vi "Video Extensometer.vi"() -> ()   [LabVIEW 2013]
uses:
  <vilib>/userdefined/High Color/IMAQdx.ctl
  <vilib>/vision/driver/IMAQdx.llb/IMAQdx Buffer Number Mode.ctl
  <vilib>/Analysis/baseanly.llb/Mean (DBL).vi
  Instance           1 30Saved   Shear-C273-with-Unload .vi
  Instance           4 30Saved   Shear-C273-with-Unload .vi
  <vilib>/vision/driver/NI_Vision_Acquisition_Software.lvlib
  <resource>/objmgr/imaqdx.rc
  <vilib>/Analysis/NI_AALBase.lvlib
panel:
  in  "Timed \nAcquisition":bool
  in  "Data \nAcquisition \nInterval (s)":dbl=1.0 min=0.1 max=60.0
  out "Image":T1(plugin-control)
  out "Time":u32
  in  "Shutter":dbl(slide)=20.0 min=0.0 max=4095.0 step=1.0 scale=4.095..4095.0 scale format="%#.0f"
  in  "Brightness":dbl(slide)=200.0 min=0.0 max=255.0 step=1.0 scale=0.0..255.0
  in  "Gain":dbl(slide)=702.0 min=350.0 max=1000.0 step=1.0 scale=350.0..1000.0
  in  "Video Mode Top":u32(ring)=47 items=["320x240 Color"=4, "640x480 Mono8"=9, "640x480 Mono16"=19, "640x480 Color"=14, "800x600 Mono8"=21, "800x600 Mono16"=27, "800x600 Color"=24, "1024x768 Mono8"=30, "1024x768 Mono16"=36, "1024x768 Color"=33, "1280x960 Mono8"=40, "1280x960 Mono16"=46, "1280x960 Color"=43, "1388x1038 Color"=47, "1388x1038 Mono"=48]
  in  "Session In Top View":T2="cam2"
  in  "Capture Current Image":bool
  in  "Begin Loading":bool
  out "Displacement (mm)":dbl
  in  "Pause":bool
  out "Crosshead Displacement":cluster{dbl[], dbl[]}(graph)
  in  "Unload \nVelocity":dbl=20.0
  in  "Unload":bool
  in  "Load Cell\nSelection":enum16{"300lb", "5lb", "50lb", "100lb"}(ring)
  in  "Distance to Travel (microns) \nup is positive":dbl=250000.0
  in  "Velocity (microns/sec)":dbl=5.0
  in  "Filename":string
  in  "Storage Directory":path=path "D:/AMS_Users_2014_2015/Michael Rossol"
  in  "Material":string
  in  "Stop":bool
  # "Top View Camera"
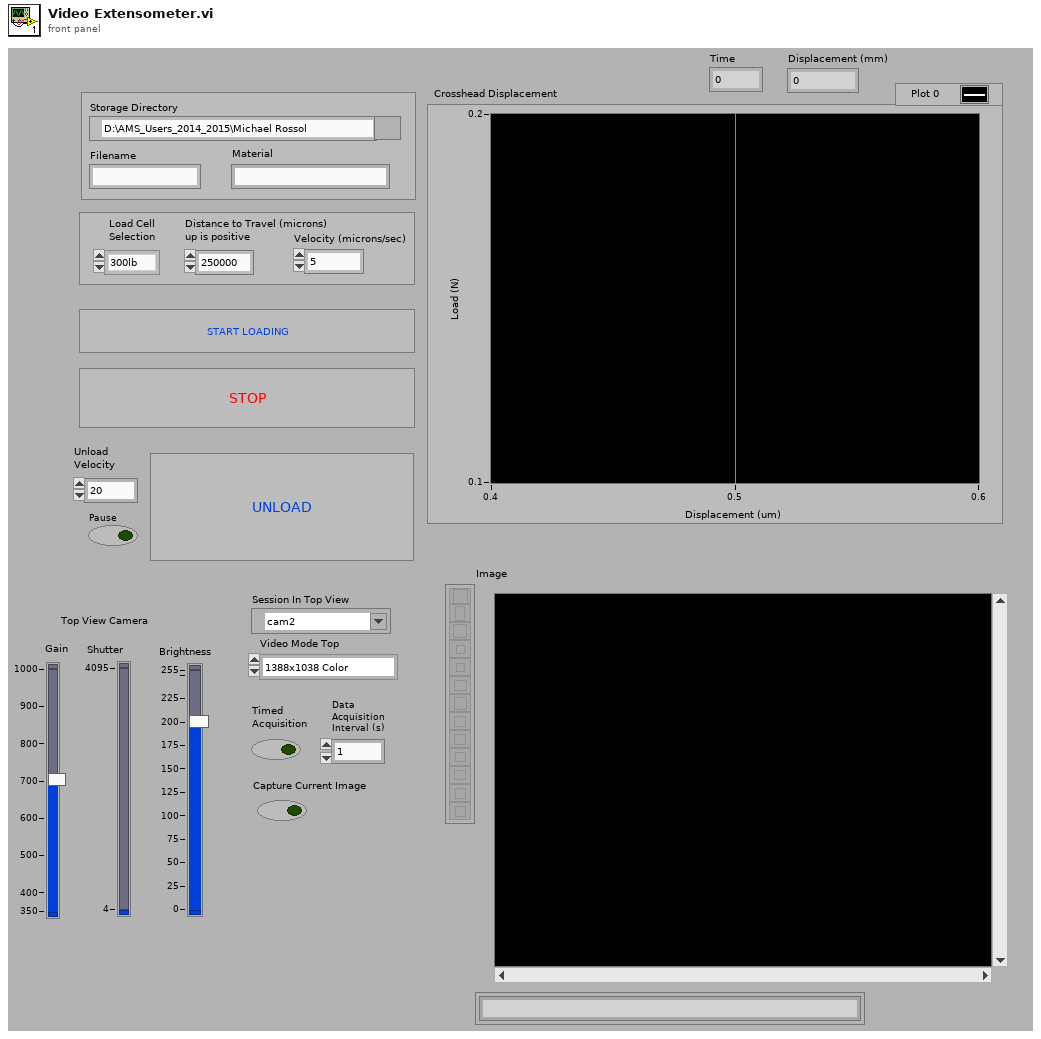
[diagram p1: front panel]
types:
  T1 = typedef "IMAQ Image.ctl" = refnum<image>
  T2 = typedef "IMAQdx.ctl" = refnum<k21>
  T3 = typedef "Image Type" = u32
  T4 = enum16{"open", "open or create", "create or replace", "create", "open (read only)"}
  T5 = typedef "NI_Vision_Acquisition_Software.lvlib/IMAQdx Buffer Number Mode.ctl" = enum32{"Next", "Last", "Buffer Number"}
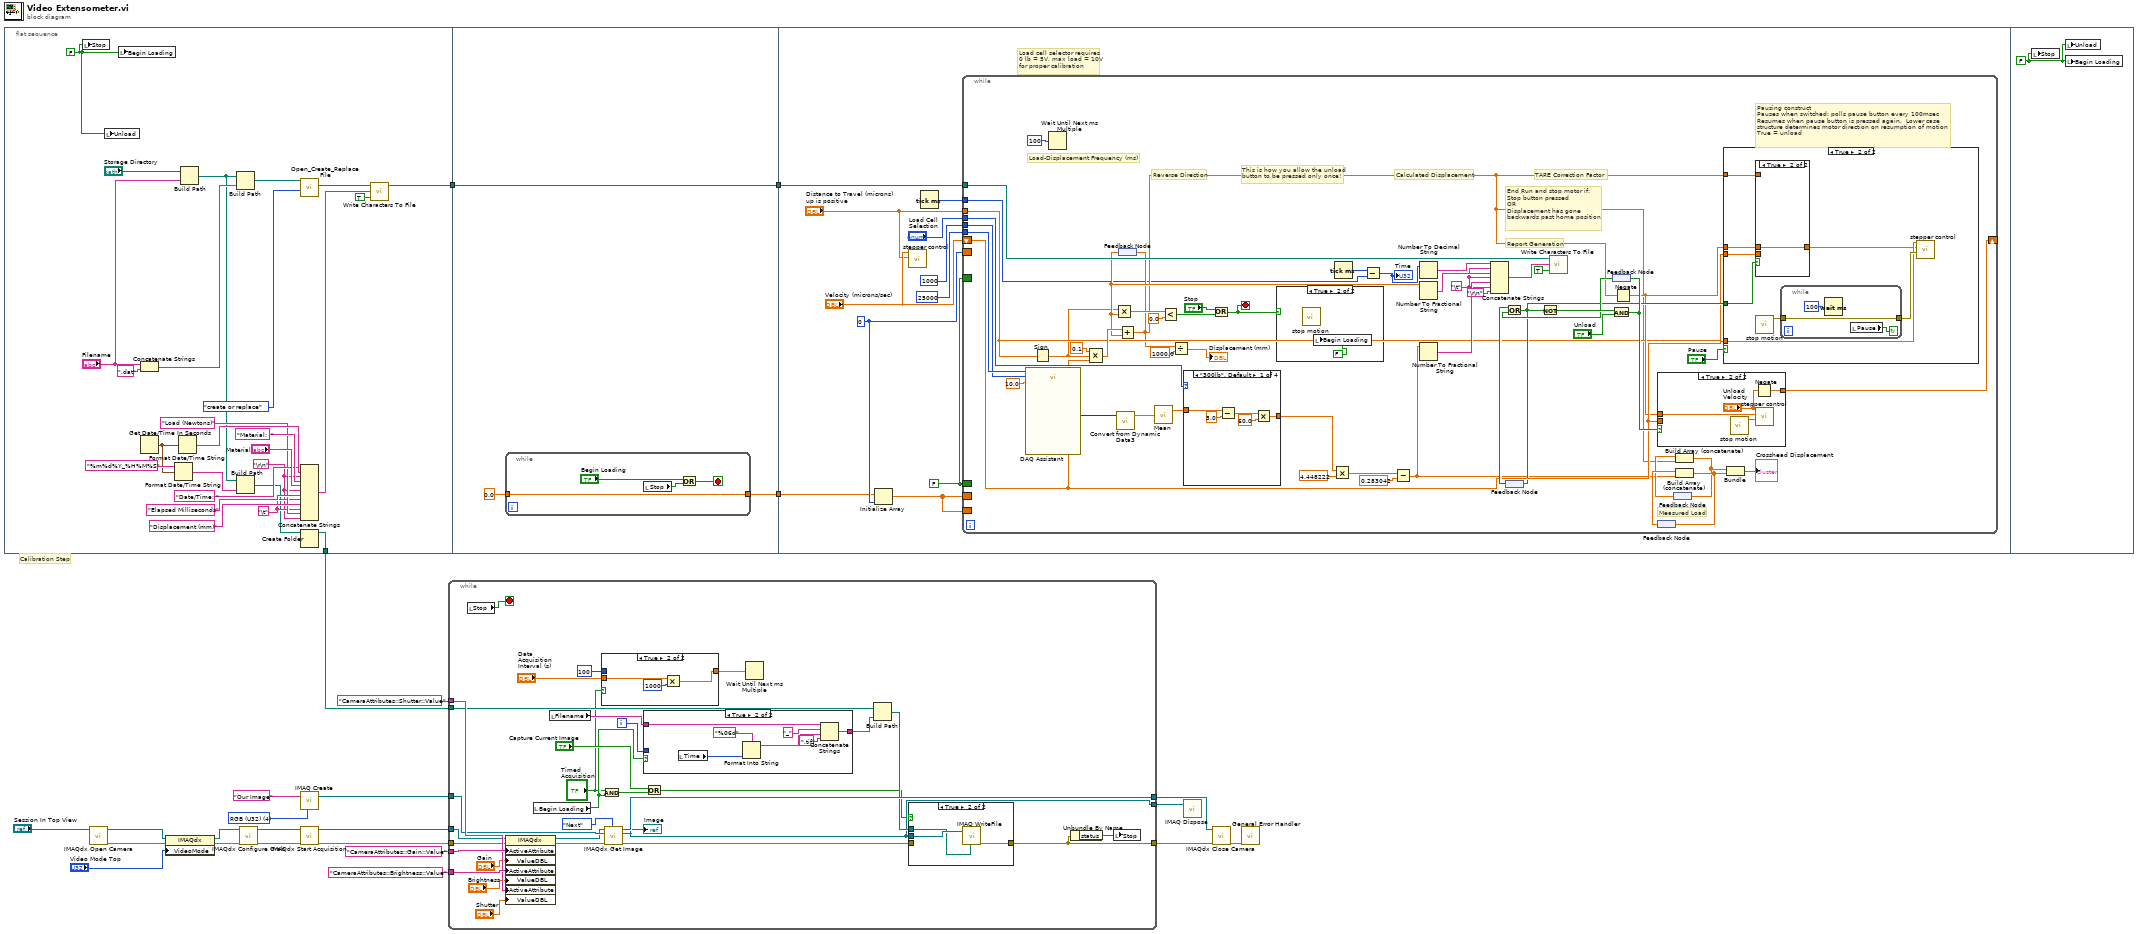
[diagram p0: block diagram]
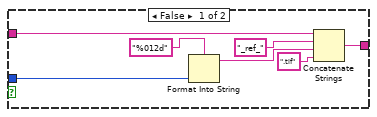
[diagram p2: hidden frame]
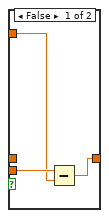
[diagram p6: hidden frame]
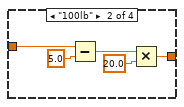
[diagram p9: hidden frame]
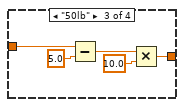
[diagram p10: hidden frame]
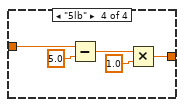
[diagram p11: hidden frame]
diagram:
  w17 = T3 4 items=["Grayscale (U8)", "Grayscale (I16)", "Grayscale (SGL)", "Complex (CSG)", "RGB (U32)", "HSL (U32)", "RGB (U64)"] ("Image Type")
  # "Calibration Step"
  n1 = flat-sequence {
    tunnel: [w41] -> w24
    tunnel: [w28] -> w1
    tunnel: w24 -> [w53]
    tunnel: [w53] -> w23
    tunnel: [w51] -> w22
    tunnel: w23 -> [w63]
    tunnel: w22 -> [w59]
    frame #0 {
      w35 = "\t"
      w25 = FALSE ("Begin Loading")
      w32 = "\r\n"
      n2 = local write "Stop"(w25) -> ()
      n3 = local write "Unload"(w25) -> ()
      n4 = local write "Begin Loading"(w25) -> ()
      n5 = Get Date/Time In Seconds() -> (seconds since 1Jan1904=w27:timestamp)
      n6 = Concatenate Strings("Filename", ".dat") -> (w47:string)
      n7 = Format Date/Time String(time format string (%c)="%m%d%Y_%H%M%S", seconds (now)=w27) -> (date/time string=w26:string)  [unwired: 1 in]
      n8 = Format Date/Time String(seconds (now)=w27) -> (date/time string=w43:string)  [unwired: 2 in]
      n9 = Build Path(base path="Storage Directory", name or relative path="Filename") -> (appended path=w30:path)
      n10 = Build Path(base path=w30, name or relative path=w47) -> (appended path=w40:path)
      n11 = Build Path(base path=w30, name or relative path=w26) -> (appended path=w29:path)
      n12 = call <vilib>:"Open_Create_Replace File.vi"("function (open:0)"=T4."create or replace", "file path"=w40) -> ("new file path"=w49:path)  [unwired: 6 in, 3 out]
      n13 = Concatenate Strings("Date/Time: ", w43, w32, "Material:  ", "Material", w32, "Elapsed Milliseconds" ("string"), w35, "Displacement (mm)" ("string"), w35, "Load (Newtons)" ("string"), w32) -> (w45:string)
      n14 = Create Folder(path (use dialog)=w29) -> (created path=w28:path)  [unwired: 2 in, 2 out]
      n15 = call <vilib>:"Write Characters To File.vi"("append to file? (new file:F)"=TRUE, "character string"=w45, "file path (dialog if empty)"=w49) -> ("new file path (Not A Path if cancelled)"=w41:path)  [unwired: 2 in]
    }
    frame #1 {
      n16 = while {
        tunnel: [w57] -> w51
        tunnel: 0.0 ("element") -> [w57]
        stop <- w55 stop-if-true
        n17 = local read "Stop"() -> (w54:bool)
        n18 = Or(x="Begin Loading", y=w54) -> (x .or. y?=w55:bool)
      }
    }
    frame #2 {
      w68 = FALSE
      w67 = 0 ("dimension size")
      # "Load cell selector requires\n0 lb = 5V, max load = 10V\nfor proper calibration"
      n19 = Initialize Array(w59, w67) -> (w66:dbl[])
      n20 = call "stepper control.vi"("Distance to Travel (microns) \nup  is positive"="Distance to Travel (microns) \nup is positive", "Velocity (microns/sec)"="Velocity (microns/sec)") -> ()  [unwired: 9 in, 1 out]
      n21 = Tick Count (ms)() -> (millisecond timer value=w58:u32)
      n22 = while {
        tunnel: "Load Cell\nSelection" -> [w119]
        tunnel: w63 -> [w109]
        shift-right: [w108] -> _
        shift-left: "Velocity (microns/sec)" -> [w93]
        tunnel: "Distance to Travel (microns) \nup is positive" -> [w90]
        border: w66 -> [_]
        border: w67 -> [_]
        border: w66 -> [_]
        border: w68 -> [_]
        border: w68 -> [_]
        tunnel: 25000 ("Sampling Rate") -> [w84]
        tunnel: 1000 ("Sampling Rate") -> [w83]
        tunnel: w58 -> [w72]
        stop <- w107 stop-if-true
        w74 = "\t"
        # "Load-Displacement Frequency (ms)"
        # "TARE Correction Factor"
        # "Pausing construct\nPauses when switched; polls pause button every 100msec\nResumes when pause button is pressed again.  Lower case\nstructure determines motor direction on resumption of motion\nTrue = unload"
        # "This is how you allow the unload\nbutton to be pressed only once!"
        # "Reverse Direction"
        # "Calculated Displacement"
        # "Measured Load"
        # "End Run and stop motor if:\nStop button pressed\nOR\nDisplacement has gone \nbackwards past home position"
        # "Report Generation"
        n23 = call "DAQ Assistant"("rate"=w84, "number of samples"=w83, "timeout (s)"=10.0 ("timeout (sec)")) -> ("data"=w85:dynamicdata)  [unwired: 14 in, 2 out]
        n24 = Sign(1:w90) -> (0:w87:dbl)
        n25 = Wait Until Next ms Multiple(millisecond multiple=100 ("Loop Timing")) -> ()  [unwired: 1 out]
        n26 = Compound Arithmetic op=MULTIPLY(0.1 ("x"), w87, w93) -> (w104:dbl)
        n27 = call "Convert from Dynamic Data3"("Dynamic Data Type"=w85) -> ("Array"=w82:dbl[])  [unwired: 3 in]
        n28 = feedback #1() -> (w88:dbl)
        n29 = Multiply(x=w87, y=w88) -> (x*y=w89:dbl)
        n30 = Add(x=w104, y=w88) -> (x+y=w77:dbl)
        n31 = feedback-in #1(w77) -> ()
        n32 = call-poly <vilib>:"Mean.vi"("X"=w82) -> ("mean"=w81:dbl)  [unwired: 1 out]
        n33 = Less?(x=w89, y=0.0) -> (x < y?=w106:bool)
        n34 = Divide(x=w77, y=1000.0 ("timeout (sec)")) -> (x/y=→"Displacement (mm)":dbl)
        n35 = case shown="\"300lb\", Default" w119 {
          tunnel: w81 -> [w144 w148 w156 w161]
          tunnel: [w146 w147 w155 w160] -> w117
          frame "300lb", Default {
            n36 = Subtract(x=w144, y=5.0) -> (x-y=w142:dbl)
            n37 = Multiply(x=w142, y=60.0) -> (x*y=w146:dbl)
          }
          frame "100lb" {
            n38 = Subtract(x=w148, y=5.0) -> (x-y=w150:dbl)
            n39 = Multiply(x=w150, y=20.0) -> (x*y=w147:dbl)
          }
          frame "50lb" {
            n40 = Subtract(x=w156, y=5.0) -> (x-y=w153:dbl)
            n41 = Multiply(x=w153, y=10.0) -> (x*y=w155:dbl)
          }
          frame "5lb" {
            n42 = Subtract(x=w161, y=5.0) -> (x-y=w158:dbl)
            n43 = Multiply(x=w158, y=1.0) -> (x*y=w160:dbl)
          }
        }
        n44 = Or(x="Stop", y=w106) -> (x .or. y?=w107:bool)
        n45 = case shown="True" w107 {
          frame False {
          }
          frame True {
            n46 = call "stop motion.vi"() -> ()  [unwired: 11 in, 1 out]
            n47 = local write "Begin Loading"(FALSE ("Begin Loading")) -> ()
          }
        }
        n48 = Multiply(x=w117, y=4.448222) -> (x*y=w80:dbl)
        n49 = Tick Count (ms)() -> (millisecond timer value=w71:u32)
        n50 = Subtract(x=w71, y=w72) -> (x-y=w70:u32)
        "Time" <- w70
        n51 = Subtract(x=w80, y=0.283042) -> (x-y=w78:dbl)
        n52 = Number To Decimal String(number=w70) -> (decimal integer string=w73:string)  [unwired: 1 in]
        n53 = Number To Fractional String(number=w88) -> (F-format string=w111:string)  [unwired: 3 in]
        n54 = Number To Fractional String(number=w78) -> (F-format string=w110:string)  [unwired: 3 in]
        n55 = Concatenate Strings(w73, w74, w111, w74, w110, w74, "\r\n") -> (w113:string)
        n56 = feedback #2() -> (w103:bool)
        n57 = call <vilib>:"Write Characters To File.vi"("append to file? (new file:F)"=TRUE, "character string"=w113, "file path (dialog if empty)"=w109) -> ()  [unwired: 2 in, 1 out]
        n58 = feedback #3() -> (w101:bool)
        n59 = Or(x=w103, y=w101) -> (x .or. y?=w92:bool)
        n60 = feedback-in #2(w92) -> ()
        n61 = Not(x=w92) -> (.not. x?=w102:bool)
        n62 = And(x=w102, y="Unload") -> (x .and. y?=w99:bool)
        n63 = feedback-in #3(w99) -> ()
        n64 = Negate(x=w77) -> (-x=w91:dbl)
        n65 = case shown="True" w99 {
          tunnel: w91 -> [_ w140]
          tunnel: [w136 w139] -> w108
          tunnel: w93 -> [w136 _]
          frame False {
          }
          frame True {
            n66 = call "stop motion.vi"() -> ("error out"=w137:errorcluster)  [unwired: 11 in]
            n67 = Negate(x="Unload \nVelocity") -> (-x=w139:dbl)
            n68 = call "stepper control.vi"("error in (no error)"=w137, "Distance to Travel (microns) \nup  is positive"=w140, "Velocity (microns/sec)"="Unload \nVelocity") -> ()  [unwired: 8 in, 1 out]
          }
        }
        n69 = feedback #4() -> (w116:dbl[])
        n70 = feedback #5() -> (w115:dbl[])
        n71 = Build Array (concatenate)(w115, w77) -> (w95:dbl[])
        n72 = feedback-in #5(w95) -> ()
        n73 = Build Array (concatenate)(w116, w78) -> (w96:dbl[])
        n74 = feedback-in #4(w96) -> ()
        n75 = case shown="True" "Pause" {
          tunnel: w93 -> [_ w127]
          tunnel: w92 -> [_ w126]
          tunnel: w91 -> [_ w125]
          tunnel: w90 -> [_ w124]
          tunnel: w77 -> [_ w122]
          frame False {
          }
          frame True {
            n76 = case shown="True" w126 {
              tunnel: w125 -> [_ w132]
              tunnel: w124 -> [w130 _]
              tunnel: [w131 w132] -> w123
              tunnel: w122 -> [w129 _]
              frame False {
                n77 = Subtract(x=w130, y=w129) -> (x-y=w131:dbl)
              }
              frame True {
              }
            }
            n78 = call "stop motion.vi"() -> ("error out"=w121:errorcluster)  [unwired: 11 in]
            n79 = while {
              tunnel: [w133] -> w128
              tunnel: w121 -> [w133]
              stop <- w135 continue-if-true
              n80 = Wait (ms)(milliseconds to wait=100 ("Loop Timing")) -> ()  [unwired: 1 out]
              n81 = local read "Pause"() -> (w135:bool)
            }
            n82 = call "stepper control.vi"("error in (no error)"=w128, "Distance to Travel (microns) \nup  is positive"=w123, "Velocity (microns/sec)"=w127) -> ()  [unwired: 8 in, 1 out]
          }
        }
        n83 = Bundle(w95, w96) -> (→"Crosshead Displacement":cluster{dbl[], dbl[]})  [unwired: 1 in]
      }
    }
    frame #3 {
      w162 = FALSE ("Stop")
      n84 = local write "Stop"(w162) -> ()
      n85 = local write "Unload"(w162) -> ()
      n86 = local write "Begin Loading"(w162) -> ()
    }
  }
  n87 = call <vilib>:"IMAQdx Open Camera.vi"("Session In"="Session In Top View") -> ("error out"=w15:errorcluster, "Session Out"=w16:T2)  [unwired: 9 in]
  n88 = property class="IMAQdx"(reference=w16, error in=w15, "VideoMode"="Video Mode Top") -> (reference out=w13:T2, error out=w14:errorcluster)
  n89 = call <vilib>:"IMAQdx Configure Grab.vi"("error in"=w14, "Session In"=w13) -> ("error out"=w11:errorcluster, "Session Out"=w12:T2)  [unwired: 8 in]
  n90 = call "IMAQ Create"("Image Name"="Our Image", "Image Type"=w17) -> ("New Image"=w8:T1)  [unwired: 3 in, 1 out]
  n91 = call <vilib>:"IMAQdx Start Acquisition.vi"("error in"=w11, "Session In"=w12) -> ("error out"=w2:errorcluster, "Session Out"=w9:T2)  [unwired: 8 in]
  n92 = while {
    tunnel: w8 -> [w190]
    tunnel: "CameraAttributes::Gain::Value" ("ActiveAttribute") -> [w193]
    tunnel: "CameraAttributes::Brightness::Value" ("ActiveAttribute") -> [w192]
    tunnel: "CameraAttributes::Shutter::Value" ("ActiveAttribute") -> [w191]
    tunnel: [w184] -> w21
    tunnel: w2 -> [w188]
    tunnel: [w182] -> w20
    tunnel: w9 -> [w185]
    tunnel: [w178] -> w3
    tunnel: w1 -> [w180]
    i -> [w170]
    stop <- w164 stop-if-true
    n93 = local read "Stop"() -> (w164:bool)
    n94 = property class="IMAQdx"(reference=w185, error in=w188, "ActiveAttribute"=w193, "ValueDBL"="Gain", "ActiveAttribute"=w192, "ValueDBL"="Brightness", "ActiveAttribute"=w191, "ValueDBL"="Shutter") -> (reference out=w187:T2, error out=w186:errorcluster)
    n95 = local read "Begin Loading"() -> (w167:bool)
    n96 = local read "Filename"() -> (w169:string)
    n97 = case shown="True" "Timed \nAcquisition" {
      tunnel: u32 100 ("y") -> [w212 _]
      tunnel: [w212 w215] -> w174
      tunnel: "Data \nAcquisition \nInterval (s)" -> [_ w214]
      frame False {
      }
      frame True {
        n98 = Multiply(x=w214, y=1000) -> (x*y=w215:dbl)
      }
    }
    n99 = And(x="Timed \nAcquisition", y=w167) -> (x .and. y?=w165:bool)
    n100 = call <vilib>:"IMAQdx Get Image.vi"("Buffer Number Mode (Next)"=IMAQdx_Buffer_Number_Mode."Next", "error in"=w186, "Image In"=w190, "Session In"=w187) -> ("error out"=w179:errorcluster, "Image Out"=w178:T1, "Session Out"=w184:T2)  [unwired: 4 in, 1 out]
    "Image" <- w178
    n101 = case shown="True" w167 {
      tunnel: [w196 w207] -> w168
      tunnel: w170 -> [w195 _]
      tunnel: w169 -> [w194 w201]
      frame False {
        n102 = Format Into String(format string="%012d", w195) -> (resulting string=w198:string)  [unwired: 2 in, 1 out]
        n103 = Concatenate Strings(w194, "_ref_" ("string"), w198, ".tif") -> (w196:string)
      }
      frame True {
        n104 = local read "Time"() -> (w204:u32)
        n105 = Format Into String(format string="%06d", w204) -> (resulting string=w203:string)  [unwired: 2 in, 1 out]
        n106 = Concatenate Strings(w201, "_" ("string"), w203, ".tif") -> (w207:string)
      }
    }
    n107 = Or(x="Capture Current Image", y=w165) -> (x .or. y?=w171:bool)
    n108 = Wait Until Next ms Multiple(millisecond multiple=w174) -> ()  [unwired: 1 out]
    n109 = Build Path(base path=w180, name or relative path=w168) -> (appended path=w183:path)
    n110 = case shown="True" w171 {
      tunnel: w178 -> [_ w211]
      tunnel: [w208 w210] -> w182
      tunnel: w183 -> [_ w209]
      tunnel: w179 -> [w208 _]
      frame False {
      }
      frame True {
        n111 = call "IMAQ WriteFile"("File Path"=w209, "Image"=w211) -> ("error out"=w210:errorcluster)  [unwired: 6 in]
      }
    }
    n112 = Unbundle By Name(w182) -> ("status"=w163:bool)
    n113 = local write "Stop"(w163) -> ()
  }
  n114 = call "IMAQ Dispose"("Image"=w3) -> ()  [unwired: 5 in, 1 out]
  n115 = call <vilib>:"IMAQdx Close Camera.vi"("error in"=w20, "Session In"=w21) -> ("error out"=w19:errorcluster)  [unwired: 9 in]
  n116 = call <vilib>:"General Error Handler.vi"("error in (no error)"=w19) -> ()  [unwired: 10 in, 5 out]
